vi "GA Set Stop Dec.vi"(8 "error in (no error)":errorcluster caption="错误输入（无错误）", 9 "decAbruptStop":dbl, 10 "decSmoothStop":dbl, 11 "nAxisNum":i16) -> (0 "error out":errorcluster caption="错误输出", 3 "function return":i32)   [LabVIEW 2015, in "GAS.lvlib"]
doc: "extern \"C\" __declspec(dllimport) int GA_SetStopDec(short nAxisNum,double decSmoothStop,double decAbruptStop);"
uses:
  <userlib>/BP_GAS/GAS.lvlib
  <userlib>/BP_GAS/GAS.dll
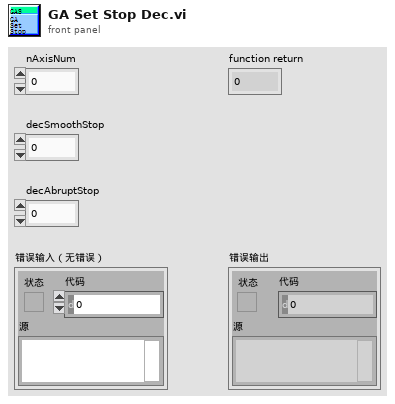
[diagram p1: front panel]
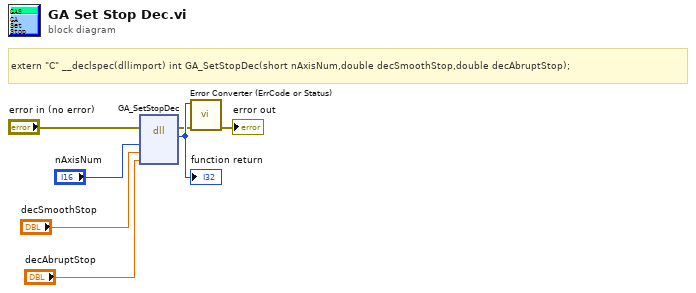
[diagram p0: block diagram]
diagram:
  # "extern \"C\" __declspec(dllimport) int GA_SetStopDec(short nAxisNum,double decSmoothStop,double decAbruptStop);"
  n1 = dll-call lib="E:/Program Files (x86)/National Instruments/LabVIEW 2015/user.lib/BP_GAS/GAS.*" fn="GA_SetStopDec"(error in="error in (no error)", "nAxisNum"="nAxisNum", "decSmoothStop"="decSmoothStop", "decAbruptStop"="decAbruptStop") -> (error out=w2:errorcluster, w7:i32)  [unwired: 5 in, 1 out]
  "function return" <- w7
  n2 = call "Error Converter (ErrCode or Status).vi"("error in (no error)"=w2, "error code"=w7) -> ("error out"=→"error out":errorcluster)  [unwired: 9 in]
